vi "set datatype.vi"(8 "error in (no error)":errorcluster, 10 "datatype":T1, 11 "JSON Helper in":refnum<class "JSON Value.lvclass">) -> (0 "error out":errorcluster, 3 "JSON Helper out":refnum<class "JSON Value.lvclass">)   [LabVIEW 2016, in "JSON Value.lvclass"]
uses:
  JSON Value.lvclass
  JSON Types.ctl
  JSON Value.lvclass/JSON Value.ctl
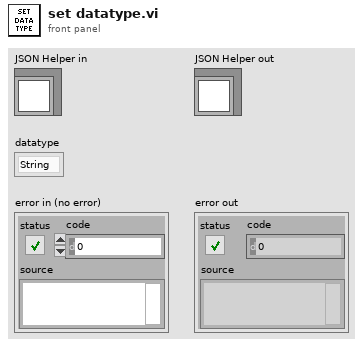
[diagram p1: front panel]
types:
  T1 = typedef "JSON Value.lvclass/JSON Types.ctl" = enum16{"String", "Numeric", "Boolean", "NULL", "Object", "Array"}
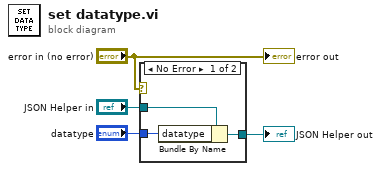
[diagram p0: block diagram]
diagram:
  n1 = case shown="No Error" "error in (no error)" {
    tunnel: "datatype" -> [w7 _]
    tunnel: [w6 w8] -> w3
    tunnel: "JSON Helper in" -> [w5 w8]
    frame No Error {
      n2 = Bundle By Name(cluster=w5, "datatype"=w7) -> (w6:refnum<class "JSON Value.lvclass">)
    }
    frame Error {
    }
  }
  "JSON Helper out" <- w3
  "error out" <- "error in (no error)"
